vi "test_Add Grouped Scalar Input Channels.vi"(8 "error in (no error)":errorcluster, 11 "TestCase in":refnum<class "FPGA Addon Adding Channel Items Unit Tests.lvclass">) -> (0 "error out":errorcluster, 3 "TestCase out":refnum<class "FPGA Addon Adding Channel Items Unit Tests.lvclass">)   [LabVIEW 2019, in "FPGA Addon Adding Channel Items Unit Tests.lvclass"]
uses:
  FPGA Addon Adding Channel Items Unit Tests.lvclass
  <vilib>/NI VeriStand/Custom Device API/Custom Device Channel.ctl
  <vilib>/NI VeriStand/Custom Device API/Custom Device Channel Type.ctl
  Addon/Addon Shared/Types/FG Action.ctl
  Addon/Addon System Explorer/Types/Channel Type.ctl
  FPGA Addon Adding Channel Items Unit Tests.lvclass/FPGA Addon Adding Channel Items Unit Tests.ctl
  Addon/Addon Shared/SubVIs/Constants.vi
  <vilib>/NI VeriStand/Custom Device Tools/Custom Device Utility Library/NI VeriStand - Search for Item by GUID.vi
  <vilib>/NI/NI VeriStand Advanced SysDef API/SysDef API/SysDef.Property.Get.vi
  <vilib>/NI/NI VeriStand Advanced SysDef API/_SubVIs/SysDef.Property.Get.Variant.vi
  <vilib>/NI/NI VeriStand Advanced SysDef API/SysDef API/SysDef.Property.Set.vi
  <vilib>/NI/NI VeriStand Advanced SysDef API/_SubVIs/SysDef.Property.Set.Variant.vi
  <vilib>/NI/NI VeriStand Advanced SysDef API/_SubVIs/SysDef.Search.GUIDs.vi
  <vilib>/addons/_JKI Toolkits/VI Tester/TestCase.llb/TestCase.lvclass
  Addon/Addon System Explorer/FPGA Addon System Explorer.lvlib
  Addon/Addon Shared/FPGA Addon Shared.lvlib
  <vilib>/NI VeriStand/Custom Device Tools/Custom Device Utility Library/Custom Device Utility Library.lvlib
  <vilib>/NI/NI VeriStand Advanced SysDef API/SysDef API/Advanced System Definition.lvlib
  <vilib>/NI VeriStand/Custom Device API/Custom Device API.lvlib
  C:/Program Files (x86)/National Instruments/LabVIEW 2019/vi.lib/addons/_JKI Toolkits/VI Tester/TestCase.llb/TestCase.lvclass
panel:
  out "GUIDs":string[](array[string])
  out "Channels":T1[](array[typedef])
  in  "remove":bool
  in  "add":bool
  out "Names":string[](array[string])
  in  "Available Registers":i32[](listbox)
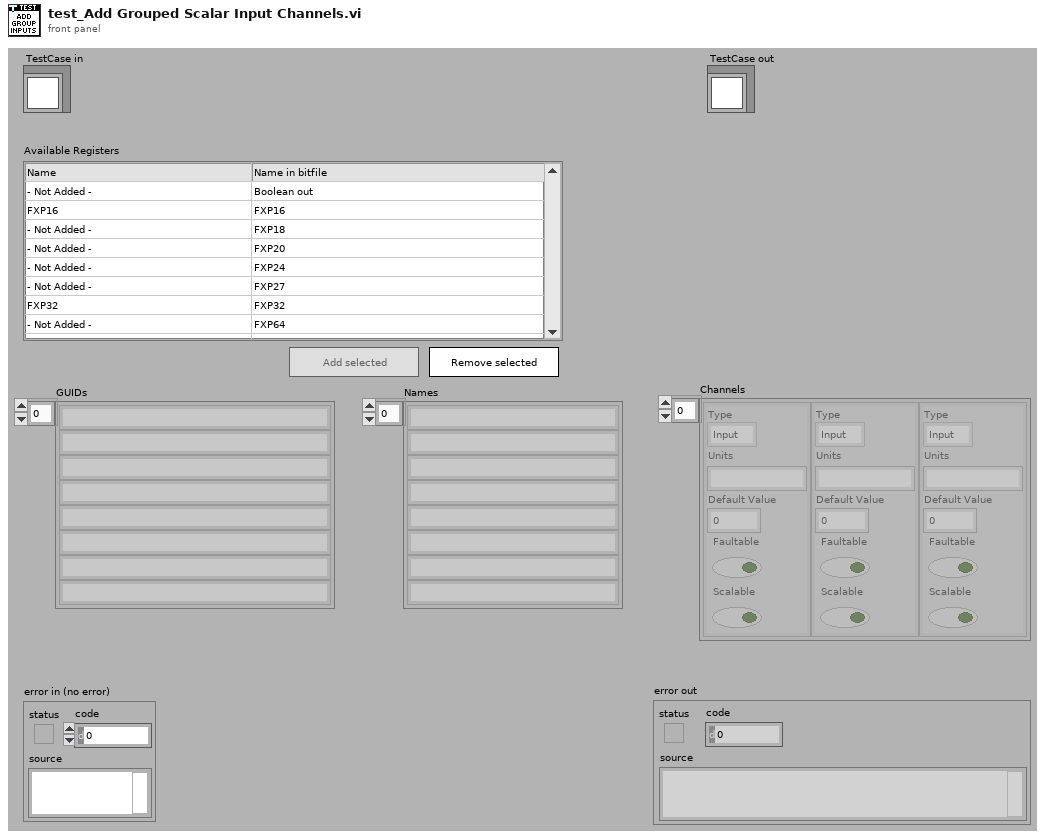
[diagram p1: front panel]
types:
  T1 = typedef "Custom Device API.lvlib/Custom Device Channel.ctl" = cluster{"Type":T2, "Units":string, "Default Value":dbl, "Faultable":bool, "Scalable":bool}
  T2 = typedef "Custom Device API.lvlib/Custom Device Channel Type.ctl" = enum16{"Input", "Output"}
  T3 = typedef "FPGA Addon System Explorer.lvlib/Channel Type.ctl" = enum16{"Write Channel", "Read Channel", "Write Waveform", "Read Waveform"}
  T4 = typedef "FPGA Addon Shared.lvlib/FG Action.ctl" = enum8{"GET", "SET"}
  T5 = typedef "Custom Device API.lvlib/Custom Device Item Ref.ctl" = u64
  T6 = typedef "FPGA Addon Shared.lvlib/Register Information.ctl" = cluster{"Name":string, "Data Type":T7, "Default Value":variant}
  T7 = typedef "FPGA Addon Shared.lvlib/Data Type.ctl" = enum8{"<Null>", "I8", "I16", "I32", "I64", "U8", "U16", "U32", "U64", "SGL", "Boolean", "Analog PWM In Settings", "Analog PWM In", "Digital PWM In Settings", "Digital PWM In", "Digital PWM Out", "Sine Out", "FXP+/-24.5", "FXP+/-16.5", "FXP+/-32.8", "FXP+/-64.32", "FXP+/-16.7", "FXP+/-20.5", "FXP+/-27.5", "FXP+/-32.16", "FXP+16.3", "FXP+18.3", "Digital Static In", "Digital Static Out", "Digital Static In Settings", "Digital WSS Out", "Quad Encoder Settings", "Quad Encoder In", "Group"}
  T8 = typedef "FPGA Addon System Explorer.lvlib/Listbox Cluster.ctl" = cluster{"add":refnum<vi>, "remove":refnum<vi>, "Listbox":refnum<vi>, "selected":i32[], "not present":i32[], "listbox text":string[][], "Section Ref":T5}
  T9 = typedef "Advanced System Definition.lvlib/TreeItem.Info.ctl" = cluster{"Name":string, "Description":string, "GUID":string, "Is Channel":bool, "Channel":T1, "Is Waveform":bool, "Waveform":T10}
  T10 = typedef "Custom Device API.lvlib/Custom Device Waveform.ctl" = cluster{"Data Type":T11, "Units":string}
  T11 = typedef "Custom Device API.lvlib/Custom Device Waveform DataType.ctl" = enum16{"Double", "Complex Double"}
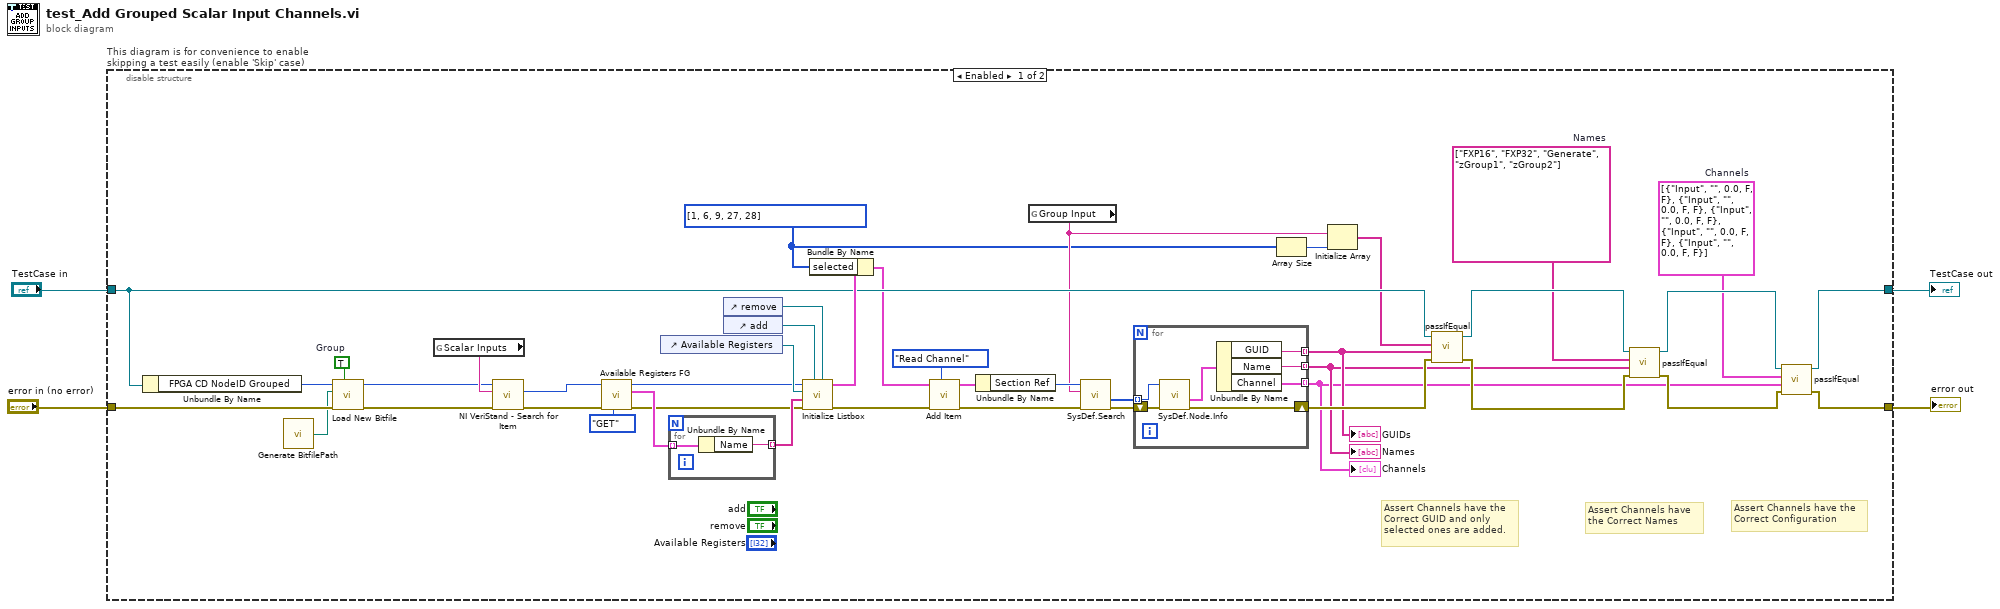
[diagram p0: block diagram]
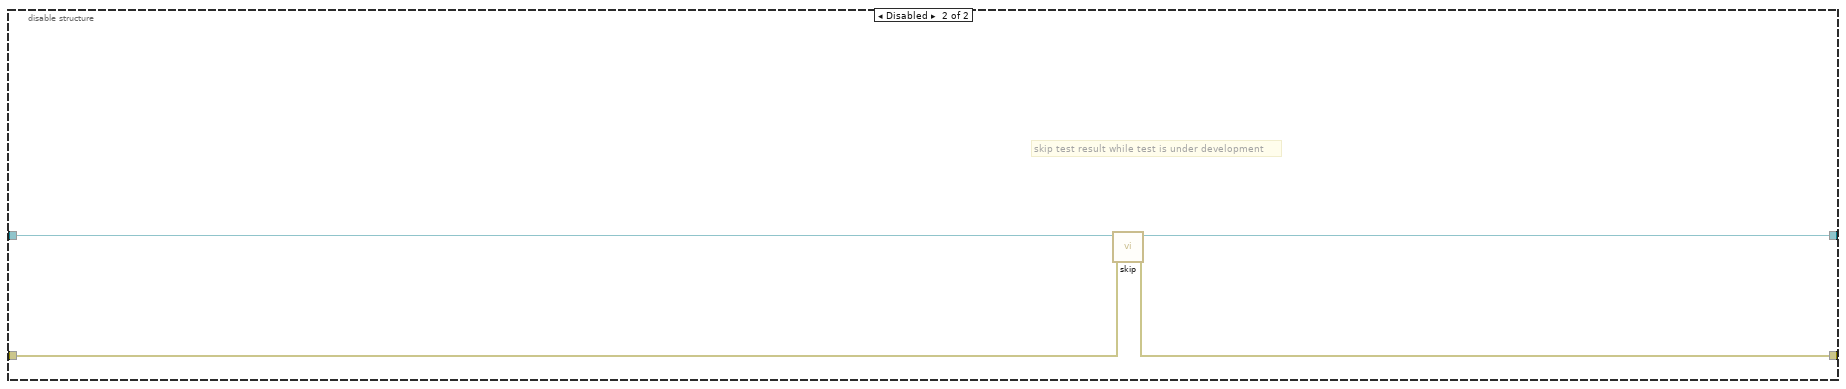
[diagram p2: hidden frame]
diagram:
  n1 = disable-structure "This diagram is for convenience to enable skipping a test easily (enable 'Skip' case)" shown="Enabled" {
    disable-tunnel: "TestCase in" -> [w27 w60]
    disable-tunnel: [w23 w58] -> w1
    disable-tunnel: [w20 w59] -> w3
    disable-tunnel: "error in (no error)" -> [w16 w57]
    frame Enabled {
      w5 = TRUE  # Group
      w18 = T1[] [{"Type"=enum."Input", "Units"="", "Default Value"=0.0, "Faultable"=FALSE, "Scalable"=FALSE}, {"Type"=enum."Input", "Units"="", "Default Value"=0.0, "Faultable"=FALSE, "Scalable"=FALSE}, {"Type"=enum."Input", "Units"="", "Default Value"=0.0, "Faultable"=FALSE, "Scalable"=FALSE}, {"Type"=enum."Input", "Units"="", "Default Value"=0.0, "Faultable"=FALSE, "Scalable"=FALSE}, {"Type"=enum."Input", "Units"="", "Default Value"=0.0, "Faultable"=FALSE, "Scalable"=FALSE}]  # Channels
      w24 = string[] ["FXP16", "FXP32", "Generate", "zGroup1", "zGroup2"]  # Names
      w7 = i32[] [1, 6, 9, 27, 28] ("selected")
      # "Assert Channels have the Correct Configuration"
      # "Assert Channels have the Correct Names"
      # "Assert Channels have the Correct GUID and only selected ones are added."
      n2 = Unbundle By Name(w27) -> ("FPGA CD NodeID Grouped"=w15:u64)
      n3 = call "Generate BitfilePath.vi"() -> ("Bitfile path"=w14:path)
      n4 = call "Load New Bitfile.vi"("Group"=w5, "error in (no error)"=w16, "NewVal"=w14, "Item Ref in"=w15) -> ("error out"=w17:errorcluster, "Section Ref out"=w13:T5)  [unwired: 6 in]
      n5 = global read "Constants.vi" "Scalar Inputs"() -> (w41:string)
      n6 = call-poly <vilib>:"NI VeriStand - Search for Item.vi"("error in"=w17, "Item GUID"=w41, "Section Ref in"=w13) -> ("error out"=w40:errorcluster, "Item Ref"=w35:T5)  [unwired: 5 in, 2 out]
      n7 = call "Available Registers FG.vi"("Action"=FG_Action."GET", "error in (no error)"=w40, "Item Ref"=w35) -> ("error out"=w39:errorcluster, "Available Registers"=w45:T6[], "Item Ref out"=w37:T5)  [unwired: 6 in]
      n8 = control-ref of="Available Registers"() -> (w47:refnum<vi>)
      n9 = for {
        tunnel: w45 -> [w49] mode=indexing
        tunnel: [w48] -> w44 mode=indexing
        n10 = Unbundle By Name(w49) -> ("Name"=w48:string)
      }
      n11 = control-ref of="remove"() -> (w32:refnum<vi>)
      n12 = control-ref of="add"() -> (w33:refnum<vi>)
      n13 = call "Initialize Listbox.vi"("remove"=w32, "add"=w33, "error in (no error)"=w39, "Names"=w44, "Listbox"=w47, "Item Ref"=w37) -> ("error out"=w38:errorcluster, "Listbox Refs"=w42:T8)  [unwired: 4 in]
      n14 = Bundle By Name(cluster=w42, "selected"=w7) -> (w11:T8)
      n15 = call "Add Item.vi"("Action"=Channel_Type."Read Channel", "error in (no error)"=w38, "Listbox Refs in"=w11) -> ("error out"=w12:errorcluster, "Listbox Refs out"=w10:T8)  [unwired: 7 in]
      n16 = Unbundle By Name(w10) -> ("Section Ref"=w34:T5)
      n17 = global read "Constants.vi" "Group Input"() -> (w8:string)
      n18 = call-poly <vilib>:"SysDef.Search.vi"("error in (no error)"=w12, "GUID"=w8, "nodeID"=w34) -> ("error out"=w36:errorcluster, "Values Out"=w31:u64[])  [unwired: 5 in, 2 out]
      n19 = for {
        tunnel: w31 -> [w52] mode=indexing
        tunnel: [w50] -> w25 mode=indexing
        tunnel: [w53] -> w19 mode=indexing
        tunnel: [w51] -> w28 mode=indexing
        shift-right: [w55] -> w29
        shift-left: w36 -> [w56]
        n20 = call <vilib>:"SysDef.Node.Info.vi"("error in (no error)"=w56, "nodeID"=w52) -> ("error out"=w55:errorcluster, "Item Info"=w54:T9)  [unwired: 6 in, 2 out]
        n21 = Unbundle By Name(w54) -> ("GUID"=w51:string, "Name"=w50:string, "Channel"=w53:T1)
      }
      "Names" <- w25
      "Channels" <- w19
      "GUIDs" <- w28
      n22 = Array Size(array=w7) -> (size(s)=w6:i32)
      n23 = Initialize Array(w8, w6) -> (w9:string[])
      n24 = call-dynamic "passIfEqual.vi"("error in (no error)"=w29, "y"=w28, "x"=w9, "TestCase in"=w27) -> ("error out"=w30:errorcluster, "TestCase out"=w26:refnum<class "FPGA Addon Adding Channel Items Unit Tests.lvclass">)  [unwired: 6 in]
      n25 = call-dynamic "passIfEqual.vi"("error in (no error)"=w30, "y"=w25, "x"=w24, "TestCase in"=w26) -> ("error out"=w21:errorcluster, "TestCase out"=w22:refnum<class "FPGA Addon Adding Channel Items Unit Tests.lvclass">)  [unwired: 6 in]
      n26 = call-dynamic "passIfEqual.vi"("error in (no error)"=w21, "y"=w19, "x"=w18, "TestCase in"=w22) -> ("error out"=w20:errorcluster, "TestCase out"=w23:refnum<class "FPGA Addon Adding Channel Items Unit Tests.lvclass">)  [unwired: 6 in]
    }
    frame Disabled {
      # "skip test result while test is under development"
      n27 = call <vilib>:"skip.vi"("error in (no error)"=w57, "TestCase in"=w60) -> ("error out"=w59:errorcluster, "TestCase out"=w58:refnum<class "FPGA Addon Adding Channel Items Unit Tests.lvclass">)  [unwired: 8 in]
    }
  }
  "error out" <- w3
  "TestCase out" <- w1
